vi "Initialize Configuration Channels.vi"(8 "error in (no error)":errorcluster, 10 "Configuration Channels":string[](array[string]), 11 "Session in":T1) -> (0 "error out":errorcluster, 3 "Session out":T1)   [LabVIEW 2017, in "NI-SWITCH Messaging.lvlib" / "NI-SWITCH Consumer.lvclass"]
uses:
  NI-SWITCH Consumer.lvclass
  <vilib>/userdefined/High Color/SLSC_Switch/nislscslSession.ctl
  <resource>/objmgr/nislscsl.rc
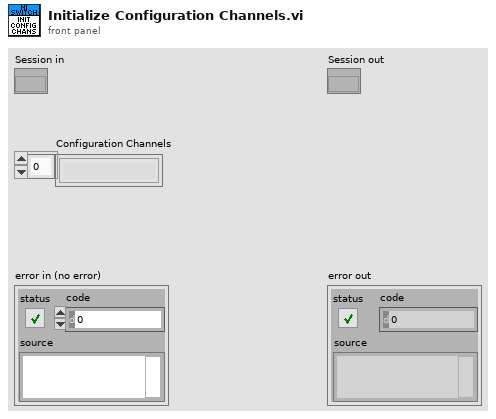
[diagram p1: front panel]
types:
  T1 = typedef "nislscslSession.ctl" = refnum<k20>
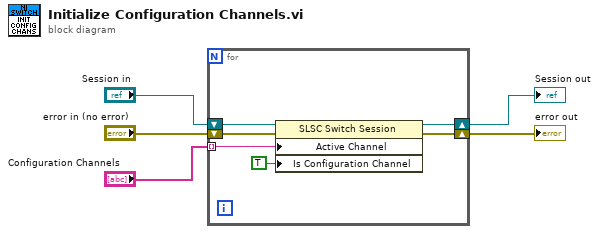
[diagram p0: block diagram]
diagram:
  n1 = for {
    shift-right: [w10] -> w5
    shift-left: "error in (no error)" -> [w11]
    shift-right: [w8] -> w3
    shift-left: "Session in" -> [w9]
    tunnel: "Configuration Channels" -> [w7] mode=indexing
    n2 = property class="SLSC Switch Session"(reference=w9, error in=w11, "Active Channel"=w7, "Is Configuration Channel"=TRUE ("Channel Configuration:Is Configuration Channel")) -> (reference out=w8:T1, error out=w10:errorcluster)
  }
  "Session out" <- w3
  "error out" <- w5
